vi "E517_All_VIs.vi"   [LabVIEW 2011]
doc: "This VI contains all high level and low level VIs valid for E-517. \nSee diagram for a survey of all E-517 high level and low level VIs. \nMenu / Browse / Show VI Hierarchy will show the file paths of the VIs. \nGlobal Variables are shown as Control as well as Indicator."
uses:
  Low Level/General command.llb/Controller names.ctl
  Low Level/Communication.llb/Available DLL interfaces.ctl
  Low Level/Communication.llb/Available DLLs.ctl
  Low Level/Communication.llb/Available interfaces.ctl
  Low Level/Communication.llb/Termination character.ctl
  Low Level/Analog control.llb/Available Analog Commands.ctl
  Low Level/Communication.llb/Global1.vi
  Low Level/General command.llb/Global2 (Array).vi
  Low Level/Communication.llb/Global DaisyChain.vi
  Low Level/Analog control.llb/Global Analog.vi
  Low Level/Support.llb/Unbunde/bundle interface clusters for PI Terminal.vi
panel:
  # "E-517 PI GCS LabVIEW driver set"
  # "This VI contains all high level and low level VIs valid for E-517. See diagram for a survey of all E-517 high \nlevel and low level VIs. Menu / Browse / Show VI Hierarchy will show the file paths of the VIs. Global \nVariables are shown as Control as well as Indicator."
types:
  T1 = enum16{"Exit VI", "Set trigger mode", "Set recordtable rate", "Set wavetable rate", "Write sine", "Read wavetable", "Read recordtable", "Enable/disable wavegen", "Set number of wavegen cycles", "Clear wavetable", "Configure data recorder", "Assign wavetable to wavegen", "Read trigger points", "Set trigger points", "Clear trigger points", "Assign axes to triggerlines", "Write ramp waveform", "Set DDL enable", "Set DDL init", "Set Start at endpoint"}[]
  T2 = typedef "Available Analog Commands.ctl" = enum16{"INITIALIZE", "VOL?", "VOL ", "CLOSE", "MOV", "POS?", "VCO", "VCO?", "WAIT_WF", "TMN?", "TMX?", "VEL", "VEL?", "SAI?", "MVR", "ERR?", "#24", "STP", "*IDN?", "#5", "STE", "DRR?", "W_Wave", "HLP?", "W/R_Wave"}
  T3 = typedef "Termination character.ctl" = enum16{"LF", "CR", "LFCR", "CRLF"}
  T4 = typedef "Available interfaces.ctl" = u16
  T5 = typedef "Available DLLs.ctl" = u16
  T6 = typedef "Available DLL interfaces.ctl" = u16
  T7 = typedef "Controller names.ctl" = enum16{"None", "Analog", "C-702", "C-843", "C-843.PM", "C-844", "C-848", "C-865", "C-866", "C-867", "C-880", "E-516", "E-517", "E-709", "E-710", "E-712", "E-725", "E-753", "E-755", "E-761", "E-816", "E-861", "F-206", "M-840", "M-850", "M-8X0", "Mercury", "Mercury_GCS"}
  T8 = cluster{"Conversion factor":dbl[], "Velocity":dbl[], "Velocity control mode":bool, "AO.Resolution":dbl, "Lower voltage limit (V)":dbl, "Upper voltage limit (V)":dbl, "AO_WF_T (s)":dbl, "AI Sample Rate":dbl, "AI Samples/Channel":i32, "Hyperbit":bool, "Offset (V)":dbl[], "Hyperbit StayOnPos":bool, "Gain (V)":dbl[], "Bit rate (Hz)":dbl, "PWM rate (Hz)":dbl, "HyperBit Password":string, "AO.MaxRate":dbl, "Conversion offset":dbl[]}[]
  T9 = cluster{"No. of devices":i32, "Port ID":i32, "Devices":string[], "Description":string}[]
  T10 = cluster{"Conn. axes":string[], "Controller name":T7}[]
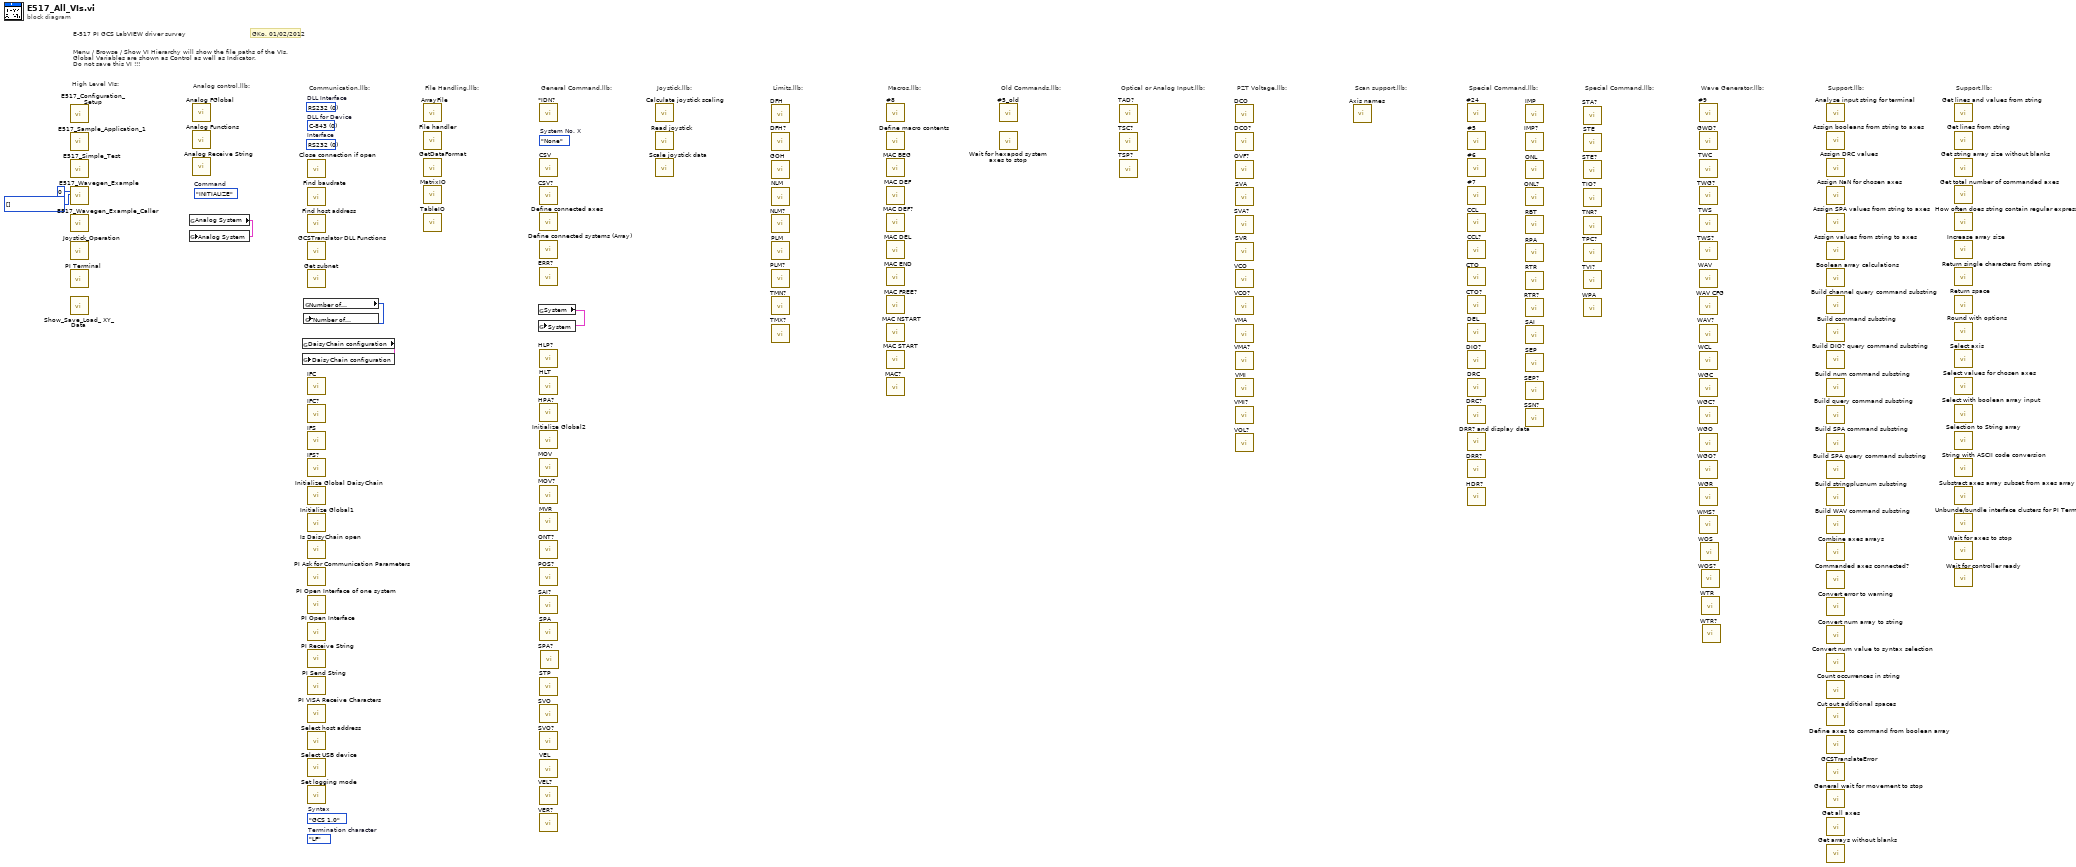
[diagram p0: block diagram]
diagram:
  w2 = T1 [] items=["Exit VI", "Set trigger mode", "Set recordtable rate", "Set wavetable rate", "Write sine", "Read wavetable", "Read recordtable", "Enable/disable wavegen", "Set number of wavegen cycles", "Clear wavetable", "Configure data recorder", "Assign wavetable to wavegen", "Read trigger points", "Set trigger points", "Clear trigger points", "Assign axes to triggerlines", "Write ramp waveform", "Set DDL enable", "Set DDL init", "Set Start at endpoint"] ("Programmatic events")
  (unwired) enum16{"GCS 1.0", "GCS 2.0"}."GCS 1.0"  # Syntax
  (unwired) Available_Analog_Commands."INITIALIZE"  # Command
  (unwired) Termination_character."LF"  # Termination character
  (unwired) T4 0 items=["RS232", "GPIB", "DLL", "TCP-IP"]  # Interface
  (unwired) T5 0 items=["C-843", "C-844", "E-710", "C-843.PM", "C-865", "E-761", "Mercury", "E-755", "E-753", "C-866", "E-712", "E-725", "E-861", "C-867", "E-517"]  # DLL for Device
  (unwired) T6 0 items=["RS232", "GPIB", "Board", "TCP-IP", "USB"]  # DLL Interface
  (unwired) Controller_names."None"  # System No. X
  # "Scan support.llb:"
  # "GKo, 01/02/2012"
  # "High Level VIs:"
  # "Analog control.llb:"
  # "Support.llb:"
  # "Wave Generator.llb:"
  # "Special Command.llb:"
  # "Support.llb:"
  # "Special Command.llb:"
  # "PZT Voltage.llb:"
  # "Optical or Analog Input.llb:"
  # "Old Commands.llb:"
  # "Macros.llb:"
  # "Limits.llb:"
  # "Joystick.llb:"
  # "General Command.llb:"
  # "File Handling.llb:"
  # "Menu / Browse / Show VI Hierarchy will show the file paths of the VIs. \nGlobal Variables are shown as Control as well as Indicator.\nDo not save this VI !!!"
  # "E-517 PI GCS LabVIEW driver survey"
  # "Communication.llb:"
  n1 = call "E517_Configuration_Setup.vi"() -> ()  [unwired: 13 in, 7 out]
  n2 = call "E517_Sample_Application_1.vi"() -> ()  [unwired: 1 out]
  n3 = call "E517_Simple_Test.vi"() -> ()  [unwired: 8 in, 12 out]
  n4 = call "E517_Wavegen_Example.vi"("# Wavegenerators"=0, "Programmatic events"=w2) -> ()  [unwired: 7 in, 11 out]
  n5 = call "E517_Wavegen_Example_Caller.vi"() -> ()  [unwired: 1 out]
  n6 = call "Joystick_Operation.vi"() -> ()  [unwired: 15 in, 5 out]
  n7 = call "PI Terminal.vi"() -> ()  [unwired: 20 out]
  n8 = call "Show_Save_Load_ XY_Data.vi"() -> ()  [unwired: 7 in, 13 out]
  n9 = global read "Global Analog.vi" "Analog System"() -> (w3:T8)
  n10 = global write "Global Analog.vi" "Analog System"(w3) -> ()
  n11 = call "Analog FGlobal.vi"() -> ()  [unwired: 3 in, 17 out]
  n12 = call "Analog Functions.vi"() -> ()  [unwired: 7 in, 13 out]
  n13 = call "Analog Receive String.vi"() -> ()  [unwired: 5 in, 15 out]
  n14 = global read "Global DaisyChain.vi" "DaisyChain configuration"() -> (w4:T9)
  n15 = global write "Global DaisyChain.vi" "DaisyChain configuration"(w4) -> ()
  n16 = global read "Global1.vi" "Number of\nsystems"() -> (w6:i32)
  n17 = global write "Global1.vi" "Number of\nsystems"(w6) -> ()
  n18 = call "Close connection if open.vi"() -> ()  [unwired: 3 in, 17 out]
  n19 = call "Find baudrate.vi"() -> ()  [unwired: 10 in, 10 out]
  n20 = call "Find host address.vi"() -> ()  [unwired: 6 in, 14 out]
  n21 = call "GCSTranslator DLL Functions.vi"() -> ()  [unwired: 7 in, 13 out]
  n22 = call "Get subnet.vi"() -> ()  [unwired: 20 out]
  n23 = call "IFC.vi"() -> ()  [unwired: 4 in, 16 out]
  n24 = call "IFC?.vi"() -> ()  [unwired: 4 in, 16 out]
  n25 = call "IFS.vi"() -> ()  [unwired: 5 in, 15 out]
  n26 = call "IFS?.vi"() -> ()  [unwired: 4 in, 16 out]
  n27 = call "Initialize Global DaisyChain.vi"() -> ()  [unwired: 2 in, 18 out]
  n28 = call "Initialize Global1.vi"() -> ()  [unwired: 2 in, 18 out]
  n29 = call "Is DaisyChain open.vi"() -> ()  [unwired: 2 in, 18 out]
  n30 = call "PI Ask for Communication Parameters.vi"() -> ()  [unwired: 20 out]
  n31 = call "PI Open Interface of one system.vi"() -> ()  [unwired: 12 in, 8 out]
  n32 = call "PI Open Interface.vi"() -> ()  [unwired: 12 in, 8 out]
  n33 = call "PI Receive String.vi"() -> ()  [unwired: 3 in, 17 out]
  n34 = call "PI Send String.vi"() -> ()  [unwired: 4 in, 16 out]
  n35 = call "PI VISA Receive Characters.vi"() -> ()  [unwired: 3 in, 17 out]
  n36 = call "Select host address.vi"() -> ()  [unwired: 6 in, 14 out]
  n37 = call "Select USB device.vi"() -> ()  [unwired: 5 in, 15 out]
  n38 = call "Set logging mode.vi"() -> ()  [unwired: 4 in, 16 out]
  n39 = call "ArrayFile.vi"() -> ()  [unwired: 20 out]
  n40 = call "File handler.vi"() -> ()  [unwired: 6 in, 14 out]
  n41 = call "GetDataFormat.vi"() -> ()  [unwired: 2 in, 18 out]
  n42 = call "MatrixIO.vi"() -> ()  [unwired: 7 in, 13 out]
  n43 = call "TableIO.vi"() -> ()  [unwired: 6 in, 14 out]
  n44 = global read "Global2 (Array).vi" "System"() -> (w5:T10)
  n45 = global write "Global2 (Array).vi" "System"(w5) -> ()
  n46 = call "*IDN?.vi"() -> ()  [unwired: 2 in, 18 out]
  n47 = call "CSV.vi"() -> ()  [unwired: 3 in, 17 out]
  n48 = call "CSV?.vi"() -> ()  [unwired: 2 in, 18 out]
  n49 = call "Define connected axes.vi"() -> ()  [unwired: 5 in, 15 out]
  n50 = call "Define connected systems (Array).vi"() -> ()  [unwired: 4 in, 16 out]
  n51 = call "ERR?.vi"() -> ()  [unwired: 2 in, 18 out]
  n52 = call "HLP?.vi"() -> ()  [unwired: 2 in, 18 out]
  n53 = call "HLT.vi"() -> ()  [unwired: 5 in, 15 out]
  n54 = call "HPA?.vi"() -> ()  [unwired: 2 in, 18 out]
  n55 = call "Initialize Global2.vi"() -> ()  [unwired: 2 in, 18 out]
  n56 = call "MOV.vi"() -> ()  [unwired: 5 in, 15 out]
  n57 = call "MOV?.vi"() -> ()  [unwired: 5 in, 15 out]
  n58 = call "MVR.vi"() -> ()  [unwired: 5 in, 15 out]
  n59 = call "ONT?.vi"() -> ()  [unwired: 5 in, 15 out]
  n60 = call "POS?.vi"() -> ()  [unwired: 5 in, 15 out]
  n61 = call "SAI?.vi"() -> ()  [unwired: 5 in, 15 out]
  n62 = call "SPA.vi"() -> ()  [unwired: 10 in, 10 out]
  n63 = call "STP.vi"() -> ()  [unwired: 5 in, 15 out]
  n64 = call "SVO.vi"() -> ()  [unwired: 5 in, 15 out]
  n65 = call "SVO?.vi"() -> ()  [unwired: 5 in, 15 out]
  n66 = call "VEL.vi"() -> ()  [unwired: 6 in, 14 out]
  n67 = call "VEL?.vi"() -> ()  [unwired: 5 in, 15 out]
  n68 = call "VER?.vi"() -> ()  [unwired: 2 in, 18 out]
  n69 = call "SPA?.vi"() -> ()  [unwired: 7 in, 13 out]
  n70 = call "Calculate joystick scaling.vi"() -> ()  [unwired: 6 in, 14 out]
  n71 = call "Read joystick.vi"() -> ()  [unwired: 2 in, 18 out]
  n72 = call "Scale joystick data.vi"() -> ()  [unwired: 8 in, 12 out]
  n73 = call "DFH.vi"() -> ()  [unwired: 5 in, 15 out]
  n74 = call "DFH?.vi"() -> ()  [unwired: 5 in, 15 out]
  n75 = call "GOH.vi"() -> ()  [unwired: 5 in, 15 out]
  n76 = call "NLM.vi"() -> ()  [unwired: 5 in, 15 out]
  n77 = call "NLM?.vi"() -> ()  [unwired: 5 in, 15 out]
  n78 = call "PLM.vi"() -> ()  [unwired: 5 in, 15 out]
  n79 = call "PLM?.vi"() -> ()  [unwired: 5 in, 15 out]
  n80 = call "TMN?.vi"() -> ()  [unwired: 5 in, 15 out]
  n81 = call "TMX?.vi"() -> ()  [unwired: 5 in, 15 out]
  n82 = call "#8.vi"() -> ()  [unwired: 2 in, 18 out]
  n83 = call "Define macro contents.vi"() -> ()  [unwired: 3 in, 17 out]
  n84 = call "MAC BEG.vi"() -> ()  [unwired: 3 in, 17 out]
  n85 = call "MAC DEF.vi"() -> ()  [unwired: 3 in, 17 out]
  n86 = call "MAC DEF?.vi"() -> ()  [unwired: 2 in, 18 out]
  n87 = call "MAC DEL.vi"() -> ()  [unwired: 4 in, 16 out]
  n88 = call "MAC END.vi"() -> ()  [unwired: 2 in, 18 out]
  n89 = call "MAC FREE?.vi"() -> ()  [unwired: 2 in, 18 out]
  n90 = call "MAC NSTART.vi"() -> ()  [unwired: 5 in, 15 out]
  n91 = call "MAC START.vi"() -> ()  [unwired: 4 in, 16 out]
  n92 = call "MAC?.vi"() -> ()  [unwired: 4 in, 16 out]
  n93 = call "#5_old.vi"() -> ()  [unwired: 2 in, 18 out]
  n94 = call "Wait for hexapod system axes to stop.vi"() -> ()  [unwired: 5 in, 15 out]
  n95 = call "TAD?.vi"() -> ()  [unwired: 5 in, 15 out]
  n96 = call "TSC?.vi"() -> ()  [unwired: 2 in, 18 out]
  n97 = call "TSP?.vi"() -> ()  [unwired: 5 in, 15 out]
  n98 = call "DCO.vi"() -> ()  [unwired: 4 in, 16 out]
  n99 = call "DCO?.vi"() -> ()  [unwired: 5 in, 15 out]
  n100 = call "OVF?.vi"() -> ()  [unwired: 5 in, 15 out]
  n101 = call "SVA.vi"() -> ()  [unwired: 5 in, 15 out]
  n102 = call "SVA?.vi"() -> ()  [unwired: 5 in, 15 out]
  n103 = call "SVR.vi"() -> ()  [unwired: 5 in, 15 out]
  n104 = call "VCO.vi"() -> ()  [unwired: 4 in, 16 out]
  n105 = call "VCO?.vi"() -> ()  [unwired: 5 in, 15 out]
  n106 = call "VMA.vi"() -> ()  [unwired: 5 in, 15 out]
  n107 = call "VMA?.vi"() -> ()  [unwired: 5 in, 15 out]
  n108 = call "VMI.vi"() -> ()  [unwired: 5 in, 15 out]
  n109 = call "VMI?.vi"() -> ()  [unwired: 5 in, 15 out]
  n110 = call "VOL?.vi"() -> ()  [unwired: 5 in, 15 out]
  n111 = call "Axis names.vi"() -> ()  [unwired: 1 in, 19 out]
  n112 = call "#24.vi"() -> ()  [unwired: 2 in, 18 out]
  n113 = call "#5.vi"() -> ()  [unwired: 2 in, 18 out]
  n114 = call "#6.vi"() -> ()  [unwired: 2 in, 18 out]
  n115 = call "#7.vi"() -> ()  [unwired: 2 in, 18 out]
  n116 = call "CCL.vi"() -> ()  [unwired: 4 in, 16 out]
  n117 = call "CCL?.vi"() -> ()  [unwired: 2 in, 18 out]
  n118 = call "CTO.vi"() -> ()  [unwired: 6 in, 14 out]
  n119 = call "CTO?.vi"() -> ()  [unwired: 5 in, 15 out]
  n120 = call "DEL.vi"() -> ()  [unwired: 3 in, 17 out]
  n121 = call "DIO?.vi"() -> ()  [unwired: 6 in, 14 out]
  n122 = call "DRC.vi"() -> ()  [unwired: 6 in, 14 out]
  n123 = call "DRC?.vi"() -> ()  [unwired: 4 in, 16 out]
  n124 = call "DRR? and display data.vi"() -> ()  [unwired: 7 in, 13 out]
  n125 = call "DRR?.vi"() -> ()  [unwired: 7 in, 13 out]
  n126 = call "HDR?.vi"() -> ()  [unwired: 3 in, 17 out]
  n127 = call "IMP.vi"() -> ()  [unwired: 5 in, 15 out]
  n128 = call "IMP?.vi"() -> ()  [unwired: 6 in, 14 out]
  n129 = call "ONL.vi"() -> ()  [unwired: 5 in, 15 out]
  n130 = call "ONL?.vi"() -> ()  [unwired: 4 in, 16 out]
  n131 = call "RBT.vi"() -> ()  [unwired: 2 in, 18 out]
  n132 = call "RPA.vi"() -> ()  [unwired: 6 in, 14 out]
  n133 = call "RTR.vi"() -> ()  [unwired: 3 in, 17 out]
  n134 = call "RTR?.vi"() -> ()  [unwired: 2 in, 18 out]
  n135 = call "SAI.vi"() -> ()  [unwired: 4 in, 16 out]
  n136 = call "SEP.vi"() -> ()  [unwired: 11 in, 9 out]
  n137 = call "SEP?.vi"() -> ()  [unwired: 7 in, 13 out]
  n138 = call "SSN?.vi"() -> ()  [unwired: 4 in, 16 out]
  n139 = call "STA?.vi"() -> ()  [unwired: 5 in, 15 out]
  n140 = call "STE.vi"() -> ()  [unwired: 6 in, 14 out]
  n141 = call "STE?.vi"() -> ()  [unwired: 6 in, 14 out]
  n142 = call "TIO?.vi"() -> ()  [unwired: 2 in, 18 out]
  n143 = call "TNR?.vi"() -> ()  [unwired: 2 in, 18 out]
  n144 = call "TPC?.vi"() -> ()  [unwired: 2 in, 18 out]
  n145 = call "TVI?.vi"() -> ()  [unwired: 3 in, 17 out]
  n146 = call "WPA.vi"() -> ()  [unwired: 7 in, 13 out]
  n147 = call "#9.vi"() -> ()  [unwired: 2 in, 18 out]
  n148 = call "GWD?.vi"() -> ()  [unwired: 6 in, 14 out]
  n149 = call "TWC.vi"() -> ()  [unwired: 2 in, 18 out]
  n150 = call "TWG?.vi"() -> ()  [unwired: 2 in, 18 out]
  n151 = call "TWS.vi"() -> ()  [unwired: 5 in, 15 out]
  n152 = call "TWS?.vi"() -> ()  [unwired: 7 in, 13 out]
  n153 = call "WAV.vi"() -> ()  [unwired: 18 in, 10 out]
  n154 = call "WAV CFG.vi"() -> ()  [unwired: 5 in, 15 out]
  n155 = call "WAV?.vi"() -> ()  [unwired: 4 in, 16 out]
  n156 = call "WCL.vi"() -> ()  [unwired: 5 in, 15 out]
  n157 = call "WGC.vi"() -> ()  [unwired: 4 in, 16 out]
  n158 = call "WGC?.vi"() -> ()  [unwired: 5 in, 15 out]
  n159 = call "WGO.vi"() -> ()  [unwired: 4 in, 16 out]
  n160 = call "WGO?.vi"() -> ()  [unwired: 5 in, 15 out]
  n161 = call "WGR.vi"() -> ()  [unwired: 2 in, 18 out]
  n162 = call "WMS?.vi"() -> ()  [unwired: 5 in, 15 out]
  n163 = call "WOS.vi"() -> ()  [unwired: 5 in, 15 out]
  n164 = call "WOS?.vi"() -> ()  [unwired: 4 in, 16 out]
  n165 = call "WTR.vi"() -> ()  [unwired: 5 in, 15 out]
  n166 = call "WTR?.vi"() -> ()  [unwired: 4 in, 16 out]
  n167 = call "Analyse input string for terminal.vi"() -> ()  [unwired: 2 in, 18 out]
  n168 = call "Assign booleans from string to axes.vi"() -> ()  [unwired: 5 in, 15 out]
  n169 = call "Assign DRC values.vi"() -> ()  [unwired: 3 in, 17 out]
  n170 = call "Assign NaN for chosen axes.vi"() -> ()  [unwired: 4 in, 16 out]
  n171 = call "Assign SPA values from string to axes.vi"() -> ()  [unwired: 7 in, 13 out]
  n172 = call "Assign values from string to axes.vi"() -> ()  [unwired: 6 in, 14 out]
  n173 = call "Boolean array calculations.vi"() -> ()  [unwired: 4 in, 16 out]
  n174 = call "Build channel query command substring.vi"() -> ()  [unwired: 7 in, 13 out]
  n175 = call "Build command substring.vi"() -> ()  [unwired: 7 in, 13 out]
  n176 = call "Build DIO? query command substring.vi"() -> ()  [unwired: 6 in, 14 out]
  n177 = call "Build num command substring.vi"() -> ()  [unwired: 3 in, 17 out]
  n178 = call "Build query command substring.vi"() -> ()  [unwired: 5 in, 15 out]
  n179 = call "Build SPA command substring.vi"() -> ()  [unwired: 10 in, 10 out]
  n180 = call "Build SPA query command substring.vi"() -> ()  [unwired: 5 in, 15 out]
  n181 = call "Build stringplusnum substring.vi"() -> ()  [unwired: 10 in, 10 out]
  n182 = call "Build WAV command substring.vi"() -> ()  [unwired: 16 in, 12 out]
  n183 = call "Combine axes arrays.vi"() -> ()  [unwired: 2 in, 18 out]
  n184 = call "Commanded axes connected?.vi"() -> ()  [unwired: 3 in, 17 out]
  n185 = call "Convert error to warning.vi"() -> ()  [unwired: 2 in, 18 out]
  n186 = call "Convert num array to string.vi"() -> ()  [unwired: 2 in, 18 out]
  n187 = call "Convert num value to syntax selection.vi"() -> ()  [unwired: 1 in, 19 out]
  n188 = call "Count occurrences in string.vi"() -> ()  [unwired: 2 in, 18 out]
  n189 = call "Cut out additional spaces.vi"() -> ()  [unwired: 2 in, 18 out]
  n190 = call "Define axes to command from boolean array.vi"() -> ()  [unwired: 4 in, 16 out]
  n191 = call "GCSTranslateError.vi"() -> ()  [unwired: 1 in, 19 out]
  n192 = call "General wait for movement to stop.vi"() -> ()  [unwired: 8 in, 12 out]
  n193 = call "Get all axes.vi"() -> ()  [unwired: 1 in, 19 out]
  n194 = call "Get arrays without blanks.vi"() -> ()  [unwired: 3 in, 17 out]
  n195 = call "Get lines and values from string.vi"() -> ()  [unwired: 2 in, 18 out]
  n196 = call "Get lines from string.vi"() -> ()  [unwired: 3 in, 17 out]
  n197 = call "Get string array size without blanks.vi"() -> ()  [unwired: 1 in, 19 out]
  n198 = call "Get total number of commanded axes.vi"() -> ()  [unwired: 2 in, 18 out]
  n199 = call "How often does string contain regular expression?.vi"() -> ()  [unwired: 2 in, 18 out]
  n200 = call "Increase array size.vi"() -> ()  [unwired: 3 in, 17 out]
  n201 = call "Return single characters from string.vi"() -> ()  [unwired: 3 in, 17 out]
  n202 = call "Return space.vi"() -> ()  [unwired: 2 in, 18 out]
  n203 = call "Round with options.vi"() -> ()  [unwired: 4 in, 16 out]
  n204 = call "Select axis.vi"() -> ()  [unwired: 2 in, 18 out]
  n205 = call "Select values for chosen axes.vi"() -> ()  [unwired: 5 in, 15 out]
  n206 = call "Select with boolean array input.vi"() -> ()  [unwired: 4 in, 16 out]
  n207 = call "Selection to String array.vi"() -> ()  [unwired: 2 in, 18 out]
  n208 = call "String with ASCII code conversion.vi"() -> ()  [unwired: 1 in, 19 out]
  n209 = call "Substract axes array subset from axes array.vi"() -> ()  [unwired: 2 in, 18 out]
  n210 = call "Unbunde/bundle interface clusters for PI Terminal.vi"() -> ()  [unwired: 6 in, 14 out]
  n211 = call "Wait for axes to stop.vi"() -> ()  [unwired: 7 in, 13 out]
  n212 = call "Wait for controller ready.vi"() -> ()  [unwired: 4 in, 16 out]
